vi "MultiChannelType_2D-Array-CXT.vi"(9 "error in":errorcluster, 11 "Array in":cxt[][](array[numeric])) -> (1 "error out":errorcluster, 2 "MultiChannelType":cxt, 3 "Array out":cxt[][](array[numeric]))   [LabVIEW 2020, in "OpenLvVision_OpenCv.lvlib"]
uses:
  <vilib>/Utility/error.llb/Error Cluster From Error Code.vi
  <vilib>/ErrorRing/Error Ring.xnode
  OpenLvVision_OpenCv.lvlib
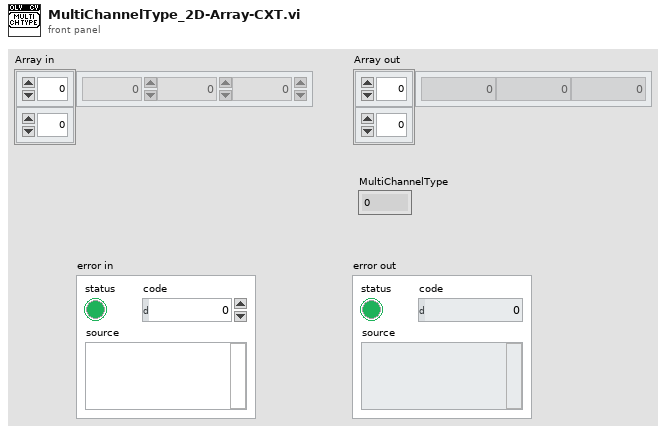
[diagram p1: front panel]
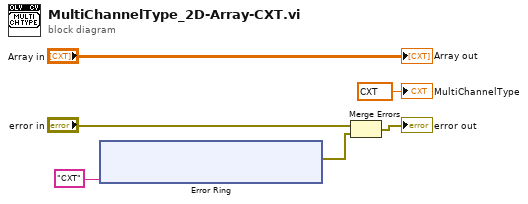
[diagram p0: block diagram]
diagram:
  n1 = xnode "Error Ring"("parameter 0"="CXT") -> ("error out"=w1:errorcluster)
  n2 = Merge Errors("error in", w1) -> (→"error out":errorcluster)
  "Array out" <- "Array in"
  "MultiChannelType" <- cxt 0.0+0.0i
